vi "SGDA-Read Data.vi"(11 "error in (no error)":errorcluster) -> (10 "AI Waveforms":dbl[][](array[numeric]), 15 "error out":errorcluster)   [LabVIEW 2020]
doc: "Sends <B>Start</B> notifier to DAQ thread to begin measurement."
uses:
  TDT VIs/TDT-Signal Bank Action.ctl
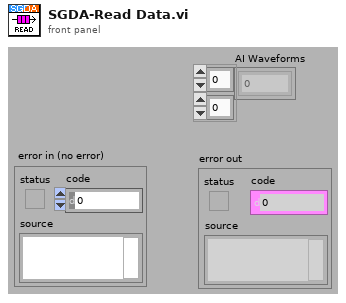
[diagram p1: front panel]
types:
  T1 = typedef "TDT-Signal Bank Action.ctl" = enum16{"Init", "Write", "Read", "Rewrite", "Reset", "Recycle", "Ramp up", "Ramp down", "Zero"}
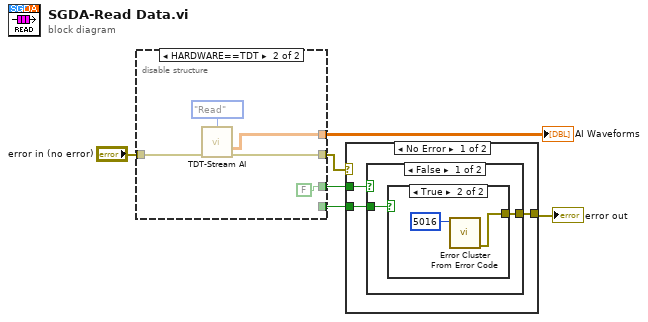
[diagram p0: block diagram]
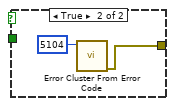
[diagram p3: hidden frame]
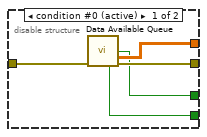
[diagram p5: hidden frame]
diagram:
  n1 = disable-structure shown="HARDWARE==TDT" {
    disable-tunnel: [w11 w16] -> w4
    disable-tunnel: "error in (no error)" -> [w10 w12]
    disable-tunnel: [w9 w15] -> w5
    disable-tunnel: [w8 FALSE ("Abort Send Data Queue")] -> w2
    disable-tunnel: [w7 _] -> w1
    frame condition #0 (active) {
      n2 = call "Data Available Queue.vi"("error in (no error)"=w10) -> ("Abort Send Data Queue"=w8:bool, "AI Waveforms"=w9:dbl[][], "Timed out"=w7:bool, "error out"=w11:errorcluster)  [unwired: 10 in, 1 out]
    }
    frame condition #1 {
      n3 = call "TDT-Stream AI.vi"("Action"=TDT-Signal_Bank_Action."Read", "error in (no error)"=w12) -> ("AI Waveforms"=w15:dbl[][], "error out"=w16:errorcluster)  [unwired: 12 in]
    }
  }
  "AI Waveforms" <- w5
  n4 = case shown="No Error" w4 {
    selector: w4 -> [_ w26]
    tunnel: [w19 w26] -> w3
    tunnel: w2 -> [w18 _]
    tunnel: w1 -> [w17 _]
    frame No Error {
      n5 = case shown="False" w18 {
        tunnel: [w20 w25] -> w19
        tunnel: w17 -> [w21 _]
        frame False {
          n6 = case shown="True" w21 {
            tunnel: [_ w22] -> w20
            frame False {
            }
            frame True {
              n7 = call <vilib>:"Error Cluster From Error Code.vi"("error code (0)"=5016) -> ("error out"=w22:errorcluster)  [unwired: 8 in]
            }
          }
        }
        frame True {
          n8 = call <vilib>:"Error Cluster From Error Code.vi"("error code (0)"=5104) -> ("error out"=w25:errorcluster)  [unwired: 8 in]
        }
      }
    }
    frame Error {
    }
  }
  "error out" <- w3
